vi "Pcre2MatchDataCreate8.vi"(8 "error in":errorcluster, 11 "OvectorCount":u32) -> (0 "error out":errorcluster, 3 "pMatchData":u64 format="%.0x")   [LabVIEW 2021, in "libpcre2-8.lvlib"]
uses:
  libpcre2-8.lvlib
  libpcre2-8-x32.dll
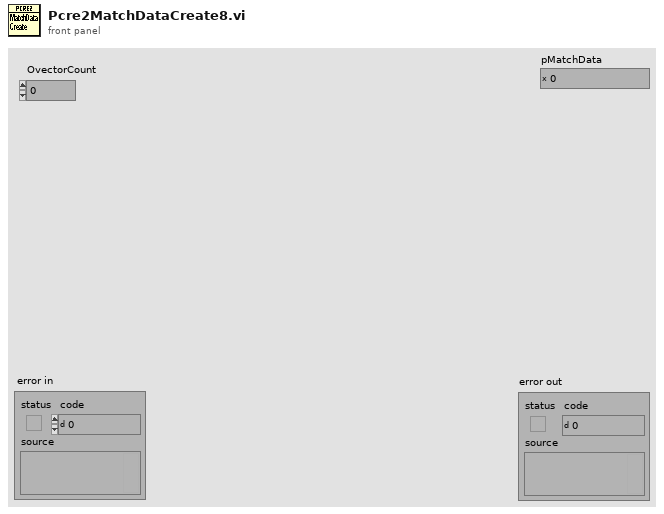
[diagram p1: front panel]
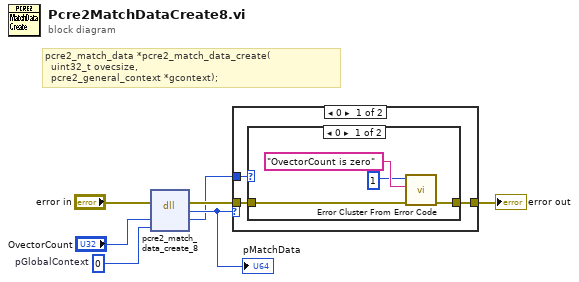
[diagram p0: block diagram]
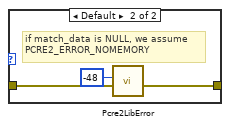
[diagram p2: hidden frame]
diagram:
  w7 = u64 0  # pGlobalContext
  # "pcre2_match_data *pcre2_match_data_create(\n  uint32_t ovecsize,\n  pcre2_general_context *gcontext);"
  n1 = dll-call lib="libpcre2-8-x*.dll" fn="pcre2_match_data_create_8"(error in="error in", "ovecsize"="OvectorCount", "gcontext"=w7) -> (error out=w2:errorcluster, "match_data"=w5:u64, "ovecsize"=w1:u32)  [unwired: 3 in, 1 out]
  "pMatchData" <- w5
  n2 = case shown="0" w5 {
    tunnel: w2 -> [w9 w18]
    tunnel: [w10 w18] -> w6
    tunnel: w1 -> [w8 _]
    frame 0 {
      n3 = case shown="0" w8 {
        tunnel: [w13 w17] -> w10
        tunnel: w9 -> [w14 w16]
        frame 0 {
          n4 = call <vilib>:"Error Cluster From Error Code.vi"("error in (no error)"=w14, "error message (\"\")"="OvectorCount is zero" ("message"), "error code (0)"=1 ("code (0)")) -> ("error out"=w13:errorcluster)  [unwired: 6 in]
        }
        frame Default {
          # "if match_data is NULL, we assume\nPCRE2_ERROR_NOMEMORY"
          n5 = call "Pcre2LibError.vi"("error in"=w16, "ErrorCode"=-48) -> ("error out"=w17:errorcluster)  [unwired: 9 in]
        }
      }
    }
    frame Default {
    }
  }
  "error out" <- w6
